vi "Elevator Launcher.vi"   [LabVIEW 2019]
uses:
  Elevator Controller/Elevator Controller/Elevator Controller.lvclass
  C:/Program Files (x86)/National Instruments/LabVIEW 2019/vi.lib/ActorFramework/Actor/Actor.lvclass
  Elevator Controller/Elevator Controller/State -Enum.ctl
  Elevator Controller/Elevator Controller Messages/Set State Msg/Set State Msg.lvclass/Set State Msg.ctl
  <vilib>/ActorFramework/Message Enqueuer/Message Enqueuer.lvclass/Message Enqueuer.ctl
  <vilib>/ActorFramework/Message Enqueuer/Enqueue.vi
  Elevator Controller/Elevator Controller Messages/Set State Msg/Set State Msg.lvclass
  C:/Program Files (x86)/National Instruments/LabVIEW 2019/vi.lib/ActorFramework/Message/Message.lvclass
  <vilib>/ActorFramework/Message Priority Queue/Priority Enqueue.vi
  <vilib>/ActorFramework/Actor/Actor.lvclass
panel:
  # "[Covers: SI1]"
types:
  T1 = typedef "Elevator Controller.lvlib/Elevator Controller.lvclass/State -Enum.ctl" = enum16{"Initial", "Wait for First Request", "Start and Move", "Analysis", "Continue Travel", "Stop at Floor", "Open and Close Door Sequence", "No request Remaining", "Emergency Call", "Terminate Process"}
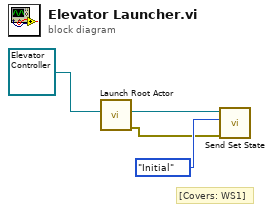
[diagram p0: block diagram]
diagram:
  # "[Covers: WS1]"
  n1 = call <vilib>:"Launch Root Actor.vi"("Actor"=refnum<class "Elevator Controller.lvclass"> refnum ("Elevator Controller.lvlib:Elevator Controller.lvclass")) -> ("error out"=w1:errorcluster, "Actor's Enqueuer"=w3:refnum<class "Message Enqueuer.lvclass">)  [unwired: 9 in]
  n2 = call "Send Set State.vi"("error in (no error)"=w1, "State"=State_-Enum."Initial", "Message Enqueuer"=w3) -> ()  [unwired: 7 in, 2 out]
